vi "Capture@ResetImaqIndex__Parameter.vi"(1 "ParamterIn":string) -> (0 "ParamterOut":string)   [LabVIEW 2019]
panel:
  in  "Index":string(combo)
  in  "ImaqName":string(combo)
  in  "Confirm":bool
  # "Capture@ResetImaqIndex $ImaqName(,$Index)"
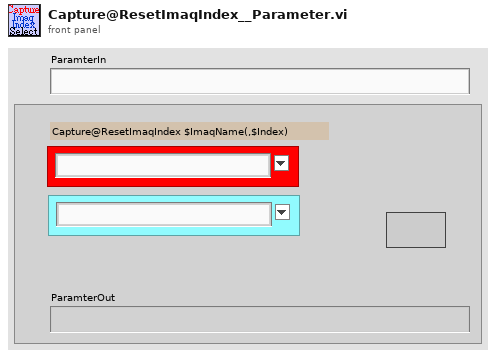
[diagram p1: front panel]
types:
  T1 = enum16{"Get", "Get&Index+1", "Insert", "Init", "Clear", "SetIndex"}
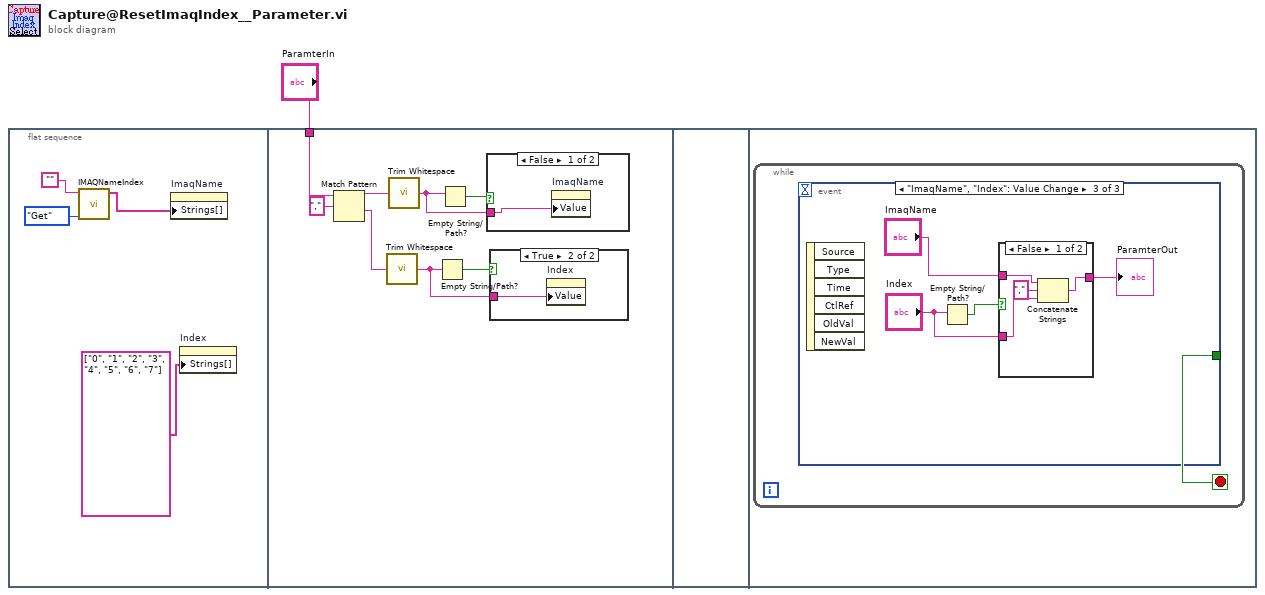
[diagram p0: block diagram]
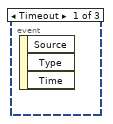
[diagram p4: hidden frame]
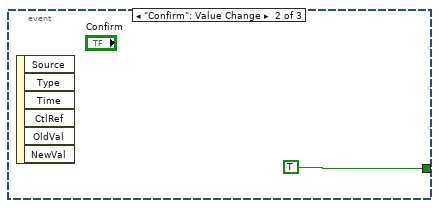
[diagram p5: hidden frame]
diagram:
  n1 = flat-sequence {
    tunnel: "ParamterIn" -> [w12]
    frame #0 {
      n2 = call "IMAQNameIndex.vi"("OP"=T1."Get", "IMAQName"="") -> ("IMAQNameList"=w2:string[])  [unwired: 2 in, 7 out]
      n3 = property on="ImaqName" class="CmbBox"("Strings[]"=w2) -> ()  [unwired: 2 in, 2 out]
      n4 = property on="Index" class="CmbBox"("Strings[]"=string[] ["0", "1", "2", "3", "4", "5", "6", "7"] ("Strings []")) -> ()  [unwired: 2 in, 2 out]
    }
    frame #1 {
      n5 = Match Pattern(string=w12, regular expression=",") -> (before substring=w9:string, after substring=w8:string)  [unwired: 1 in, 2 out]
      n6 = call <vilib>:"Trim Whitespace.vi"("string"=w8) -> ("trimmed string"=w6:string)  [unwired: 1 in]
      n7 = call <vilib>:"Trim Whitespace.vi"("string"=w9) -> ("trimmed string"=w10:string)  [unwired: 1 in]
      n8 = Empty String/Path?(string/path=w6) -> (empty?=w7:bool)
      n9 = Empty String/Path?(string/path=w10) -> (empty?=w13:bool)
      n10 = case shown="False" w13 {
        tunnel: w10 -> [w15 _]
        frame False {
          n11 = property on="ImaqName" class="CmbBox"("Value"=w15) -> ()  [unwired: 2 in, 2 out]
        }
        frame True {
        }
      }
      n12 = case shown="True" w7 {
        tunnel: w6 -> [_ w14]
        frame False {
        }
        frame True {
          n13 = property on="Index" class="CmbBox"("Value"=w14) -> ()  [unwired: 2 in, 2 out]
        }
      }
    }
    frame #2 {
    }
    frame #3 {
      n14 = while {
        stop <- w16 stop-if-true
        n15 = event shown="[2] \"ImaqName\", \"Index\": Value Change" {
          selector: _ -> [_ _ _]
          dyn-events: _ -> [_ _ _]
          timeout: _ -> [_ _ _]
          tunnel: [_ TRUE _] -> w16
          event Timeout {
            n16 = event-data() -> ()  [unwired: 1 in, 3 out]
          }
          event "Confirm": Value Change {
            n17 = event-data() -> ()  [unwired: 1 in, 6 out]
          }
          event "ImaqName", "Index": Value Change {
            n18 = event-data() -> ()  [unwired: 1 in, 6 out]
            n19 = Empty String/Path?(string/path="Index") -> (empty?=w21:bool)
            n20 = case shown="False" w21 {
              tunnel: [w22 w26] -> w19
              tunnel: "ImaqName" -> [w25 w26]
              tunnel: "Index" -> [w24 _]
              frame False {
                n21 = Concatenate Strings(w25, "," ("string"), w24) -> (w22:string)
              }
              frame True {
              }
            }
            "ParamterOut" <- w19
          }
        }
      }
    }
  }
